vi "CheckParameters.vi"(8 "error in (no error)":errorcluster, 10 "Parameters":u32[](array[numeric]), 11 "Surge in":refnum<class "Surge.lvclass">) -> (0 "error out":errorcluster, 3 "Surge out":refnum<class "Surge.lvclass">)   [LabVIEW 2013, in "Surge.lvclass"]
uses:
  Surge.lvclass
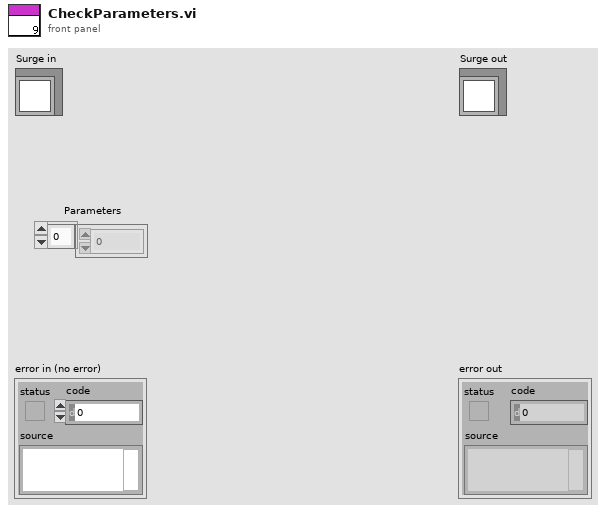
[diagram p1: front panel]
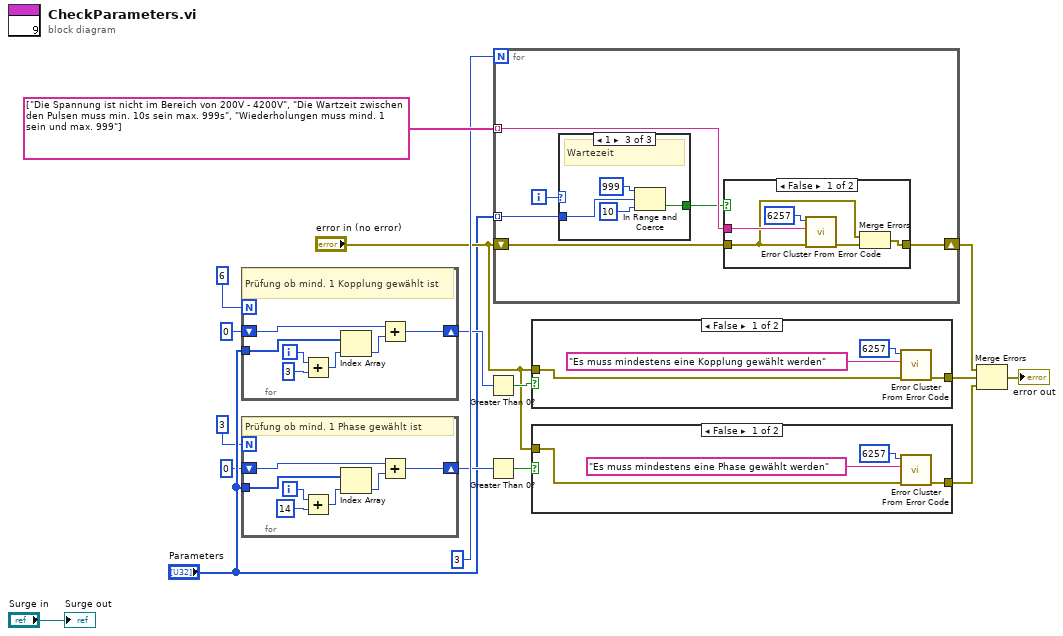
[diagram p0: block diagram]
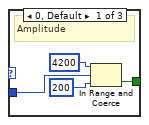
[diagram p5: hidden frame]
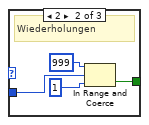
[diagram p6: hidden frame]
diagram:
  n1 = for "For-Schleife" {
    N: 6 -> [_]
    tunnel: "Parameters" -> [w22]
    shift-right: [w19] -> w13
    shift-left: u32 0 -> [w18]
    i -> [w24]
    # "Prüfung ob mind. 1 Kopplung gewählt ist"
    n2 = Add(x=w24, y=3) -> (x+y=w21:i32)
    n3 = Index Array(array=w22, index=w21) -> (element=w20:u32)
    n4 = Add(x=w18, y=w20) -> (x+y=w19:u32)
  }
  n5 = for "For-Schleife" {
    N: 3 -> [_]
    tunnel: "Parameters" -> [w29]
    shift-right: [w26] -> w8
    shift-left: u32 0 -> [w25]
    i -> [w31]
    # "Prüfung ob mind. 1 Phase gewählt ist"
    n6 = Add(x=w31, y=14) -> (x+y=w28:i32)
    n7 = Index Array(array=w29, index=w28) -> (element=w27:u32)
    n8 = Add(x=w25, y=w27) -> (x+y=w26:u32)
  }
  n9 = Greater Than 0?(x=w13) -> (x > 0?=w12:bool)
  n10 = Greater Than 0?(x=w8) -> (x > 0?=w9:bool)
  n11 = for {
    N: 3 -> [_]
    tunnel: "Parameters" -> [w37] mode=indexing
    tunnel: string[] ["Die Spannung ist nicht im Bereich von 200V - 4200V", "Die Wartzeit zwischen den Pulsen muss min. 10s sein max. 999s", "Wiederholungen muss mind. 1 sein und max. 999"] -> [w35] mode=indexing
    shift-right: [w33] -> w11
    shift-left: "error in (no error)" -> [w34]
    i -> [w36]
    n12 = case shown="1" w36 {
      tunnel: w37 -> [w47 w51 w55]
      tunnel: [w44 w48 w52] -> w32
      frame 0, Default {
        # "Amplitude"
        n13 = In Range and Coerce(upper limit=u32 4200 ("Obergrenze"), x=w47, lower limit=u32 200 ("Untergrenze")) -> (In Range?=w44:bool)  [unwired: 1 out]
      }
      frame 2 {
        # "Wiederholungen"
        n14 = In Range and Coerce(upper limit=u32 999 ("Obergrenze"), x=w51, lower limit=u32 1 ("Untergrenze")) -> (In Range?=w48:bool)  [unwired: 1 out]
      }
      frame 1 {
        # "Wartezeit"
        n15 = In Range and Coerce(upper limit=u32 999 ("Obergrenze"), x=w55, lower limit=u32 10 ("Untergrenze")) -> (In Range?=w52:bool)  [unwired: 1 out]
      }
    }
    n16 = case shown="False" w32 {
      tunnel: w35 -> [w42 _]
      tunnel: w34 -> [w40 w43]
      tunnel: [w38 w43] -> w33
      frame False {
        n17 = call <vilib>:"Error Cluster From Error Code.vi"("error in (no error)"=w40, "error message (\"\")"=w42, "error code (0)"=6257) -> ("error out"=w39:errorcluster)  [unwired: 6 in]
        n18 = Merge Errors(w40, w39) -> (w38:errorcluster)
      }
      frame True {
      }
    }
  }
  n19 = case shown="False" w12 {
    tunnel: "error in (no error)" -> [w58 w60]
    tunnel: [w57 w60] -> w10
    frame False {
      n20 = call <vilib>:"Error Cluster From Error Code.vi"("error in (no error)"=w58, "error message (\"\")"="Es muss mindestens eine Kopplung gewählt werden" ("error message (\"\")"), "error code (0)"=6257) -> ("error out"=w57:errorcluster)  [unwired: 6 in]
    }
    frame True {
    }
  }
  n21 = case shown="False" w9 {
    tunnel: "error in (no error)" -> [w63 w65]
    tunnel: [w62 w65] -> w4
    frame False {
      n22 = call <vilib>:"Error Cluster From Error Code.vi"("error in (no error)"=w63, "error message (\"\")"="Es muss mindestens eine Phase gewählt werden" ("error message (\"\")"), "error code (0)"=6257) -> ("error out"=w62:errorcluster)  [unwired: 6 in]
    }
    frame True {
    }
  }
  n23 = Merge Errors(w11, w10, w4) -> (→"error out":errorcluster)
  "Surge out" <- "Surge in"
